vi "svx_SC Line Attribute.vi"(0 "attribute":variant) -> (14 "probe angle X":u32, 15 "probe angle Y":u32, 16 "rotating direction":u16, 17 "x-axis selection":string, 18 "pair":string)   [LabVIEW 2017, in "SVX SC Line.xctl"]
uses:
  <vilib>/addons/_XControls/Shaft Centerline/SVX SC Line.xctl
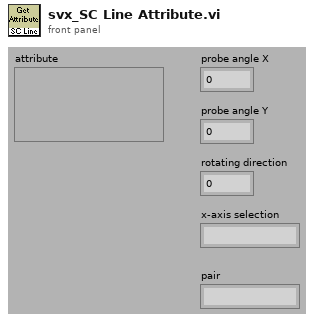
[diagram p1: front panel]
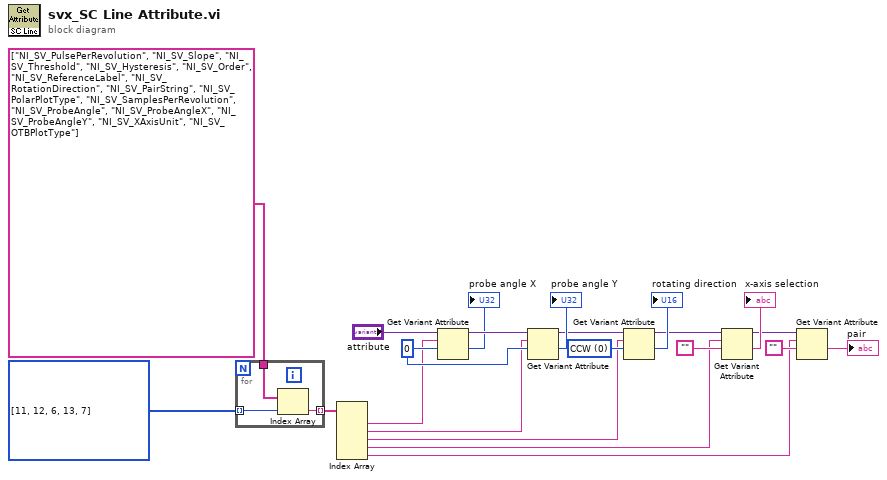
[diagram p0: block diagram]
diagram:
  w7 = u16[] [11, 12, 6, 13, 7] items=["Pulse / Revolution", "Slope", "Threshold", "Hysteresis", "Order", "Reference Label", "Rotation Direction", "Pair String", "Polar Plot Type", "Sample Per Revolution", "Probe Angle", "Probe Angle X", "Probe Angle Y", "X Axis Unit", "OTB Plot Type"]
  w16 = u16 0 items=["CCW", "CW"] ("shaft rotating direction")
  w21 = u32 0 ("probe angles X")
  n1 = for {
    tunnel: string[] ["NI_SV_PulsePerRevolution", "NI_SV_Slope", "NI_SV_Threshold", "NI_SV_Hysteresis", "NI_SV_Order", "NI_SV_ReferenceLabel", "NI_SV_RotationDirection", "NI_SV_PairString", "NI_SV_PolarPlotType", "NI_SV_SamplesPerRevolution", "NI_SV_ProbeAngle", "NI_SV_ProbeAngleX", "NI_SV_ProbeAngleY", "NI_SV_XAxisUnit", "NI_SV_OTBPlotType"] -> [w25]
    tunnel: [w24] -> w6 mode=indexing
    tunnel: w7 -> [w23] mode=indexing
    n2 = Index Array(array=w25, index=w23) -> (element=w24:string)
  }
  n3 = Index Array(array=w6) -> (element #1=w5:string, element #2=w4:string, element #3=w3:string, element #4=w2:string, element #5=w1:string)  [unwired: 5 in]
  n4 = Get Variant Attribute(Variant="attribute", name=w5, default value (empty Variant)=w21) -> (duplicate Variant=w22:variant, value=→"probe angle X":u32)  [unwired: 1 in, 2 out]
  n5 = Get Variant Attribute(Variant=w22, name=w4, default value (empty Variant)=w21) -> (duplicate Variant=w17:variant, value=→"probe angle Y":u32)  [unwired: 1 in, 2 out]
  n6 = Get Variant Attribute(Variant=w17, name=w3, default value (empty Variant)=w16) -> (duplicate Variant=w13:variant, value=→"rotating direction":u16)  [unwired: 1 in, 2 out]
  n7 = Get Variant Attribute(Variant=w13, name=w2, default value (empty Variant)="") -> (duplicate Variant=w12:variant, value=→"x-axis selection":string)  [unwired: 1 in, 2 out]
  n8 = Get Variant Attribute(Variant=w12, name=w1, default value (empty Variant)="") -> (value=→"pair":string)  [unwired: 1 in, 3 out]
